vi "Calculate Pot Value For Arm at Zero Degrees.vi"(1 "potValue":dbl, 2 "arm Angle (degrees)":dbl=0.4134002775260688) -> (0 "pottValueForArmAtZeroDegrees":sgl)   [LabVIEW 2020]
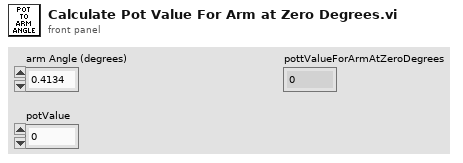
[diagram p1: front panel]
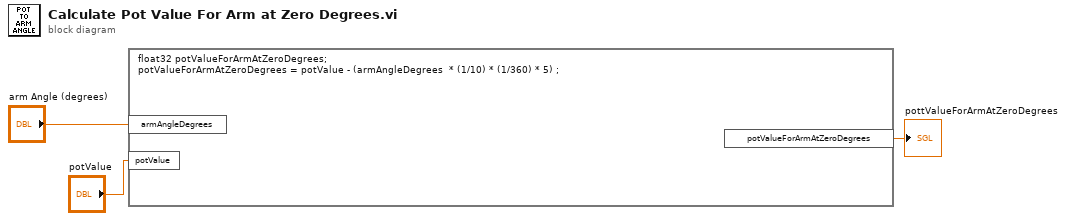
[diagram p0: block diagram]
diagram:
  n1 = formula code="float32 potValueForArmAtZeroDegrees;\npotValueForArmAtZeroDegrees = potValue - (armAngleDegrees  * (1/10) * (1/360) * 5) ;"("potValue"="potValue", "armAngleDegrees"="arm Angle (degrees)") -> ("potValueForArmAtZeroDegrees"=→"pottValueForArmAtZeroDegrees":sgl)
